vi "On Compile - Group Hardware Channels by Message Type.vi"(8 "error in":errorcluster, 11 "hardware channel data":T2[](array[typedef]) {"labels settings for RT"."Label Timestamp Channel Data Reference" format="%.0x"; "labels settings for RT"."Word Initial Raw Value" format="%032.0f"; "labels settings for RT"."Label Disable/Trigger Channel Reference" format="%.0x"; "labels settings for RT"."parameter driver data"."Tx parameter refs" format="%.0x"; "labels settings for RT"."SDI" format="%02b"; "labels settings for RT"."label" format="%.0o"}) -> (0 "error out":errorcluster, 3 "hardware channel data by transfer type":T10(array[cluster]) {"hardware channel data"."labels settings for RT"."Label Timestamp Channel Data Reference" format="%.0x"; "hardware channel data"."labels settings for RT"."Word Initial Raw Value" format="%032.0f"; "hardware channel data"."labels settings for RT"."Label Disable/Trigger Channel Reference" format="%.0x"; "hardware channel data"."labels settings for RT"."parameter driver data"."Tx parameter refs" format="%.0x"; "hardware channel data"."labels settings for RT"."SDI" format="%02b"; "hardware channel data"."labels settings for RT"."label" format="%.0o"; "Outgoing Channels" format="%.0x"; "ReadWrite Channels" format="%.0x"})   [LabVIEW 2020, in "AIM ARINC 429 System Explorer.lvlib" / "Implementation.lvlib"]
uses:
  Implementation.lvlib
  Shared/RT Hardware Channel Settings.ctl
  Shared/RT Label Settings.ctl
  Shared/Label.ctl
  Shared/RT Parameters.ctl
  Shared/Parameter Definition.ctl
  <vilib>/NI/NI VeriStand Encoding and Decoding/Encoding.ctl
  <vilib>/NI VeriStand/Custom Device API/Custom Device Item Ref.ctl
  Shared/Transfer Type.ctl
  <vilib>/NI VeriStand/Custom Device API/Data Reference.ctl
  <vilib>/NI VeriStand/Custom Device API/Custom Device API.lvlib
  <vilib>/NI/NI VeriStand Encoding and Decoding/Encoding and Decoding.lvlib
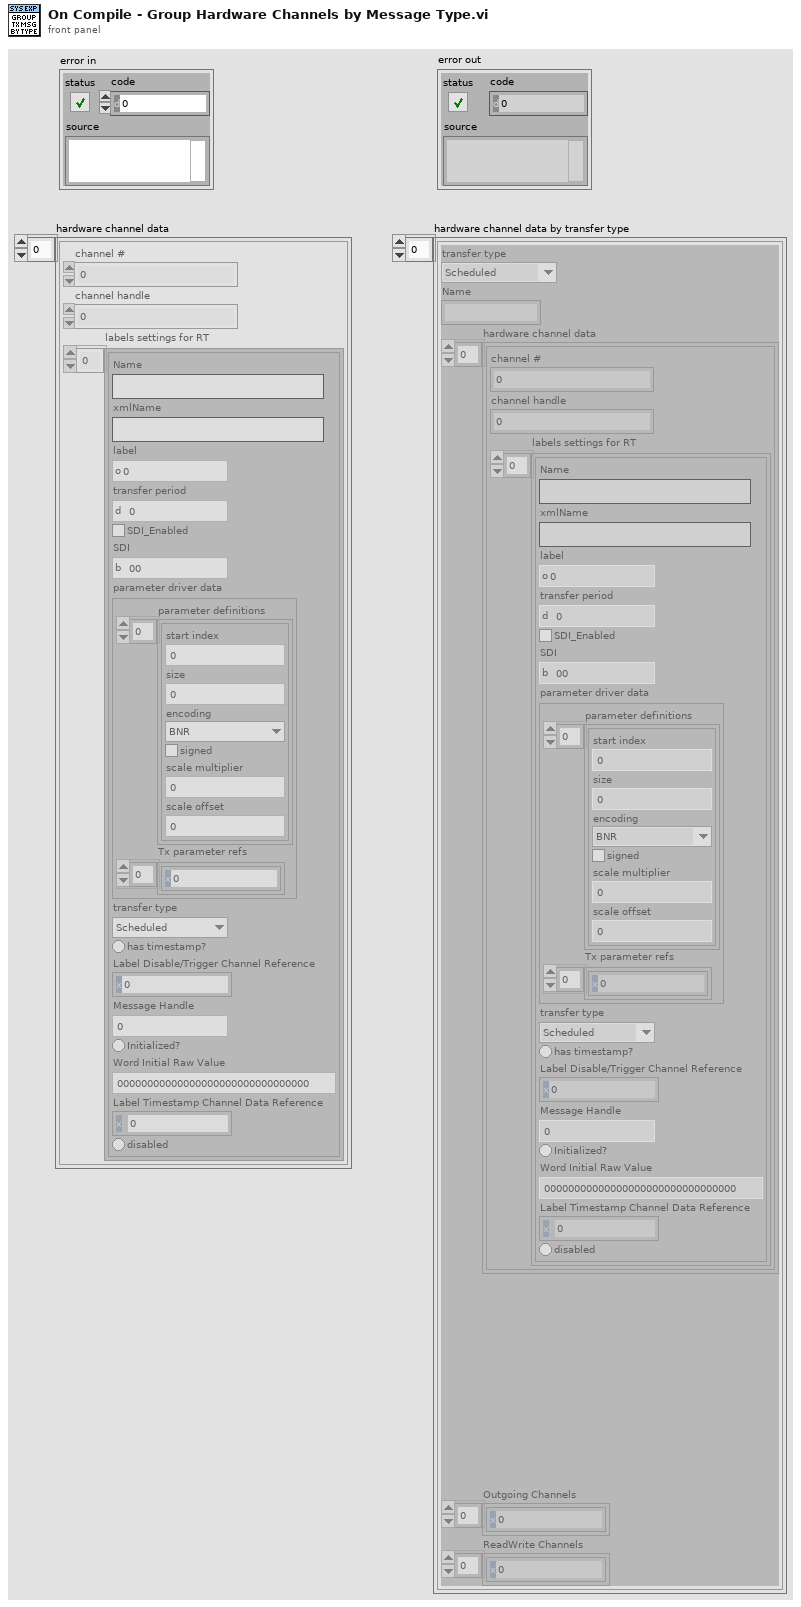
[diagram p1: front panel]
types:
  T1 = typedef "Transfer Type.ctl" = enum16{"Scheduled", "Acyclic", "Block", "Strobe"}
  T2 = typedef "RT Hardware Channel Settings.ctl" = cluster{"channel #":u16, "channel handle":u64, "labels settings for RT":T3[]}
  T3 = typedef "RT Label Settings.ctl" = cluster{"Name":string, "xmlName":string, "label":T4, "transfer period":u32, "SDI_Enabled":bool, "SDI":u8, "parameter driver data":T5, "transfer type":T1, "has timestamp?":bool, "Label Disable/Trigger Channel Reference":T8, "Message Handle":u64, "Initialized?":bool, "Word Initial Raw Value":u32, "Label Timestamp Channel Data Reference":T9, "disabled":bool}
  T4 = typedef "Label.ctl" = u8
  T5 = typedef "RT Parameters.ctl" = cluster{"parameter definitions":T6[], "Tx parameter refs":T8[]}
  T6 = typedef "Parameter Definition.ctl" = cluster{"start index":i32, "size":i32, "encoding":T7, "signed":bool, "scale multiplier":dbl, "scale offset":dbl}
  T7 = typedef "Encoding and Decoding.lvlib/Encoding.ctl" = enum16{"BNR", "BCD", "Discrete"}
  T8 = typedef "Custom Device API.lvlib/Custom Device Item Ref.ctl" = u64
  T9 = typedef "Custom Device API.lvlib/Data Reference.ctl" = i32
  T10 = cluster{"transfer type":T1, "Name":string, "hardware channel data":T2[], "Outgoing Channels":T8[], "ReadWrite Channels":T8[]}[]
  T11 = cluster{"transfer type":T1, "Name":string, "hardware channel data":T2[], "Outgoing Channels":T8[], "ReadWrite Channels":T8[]}
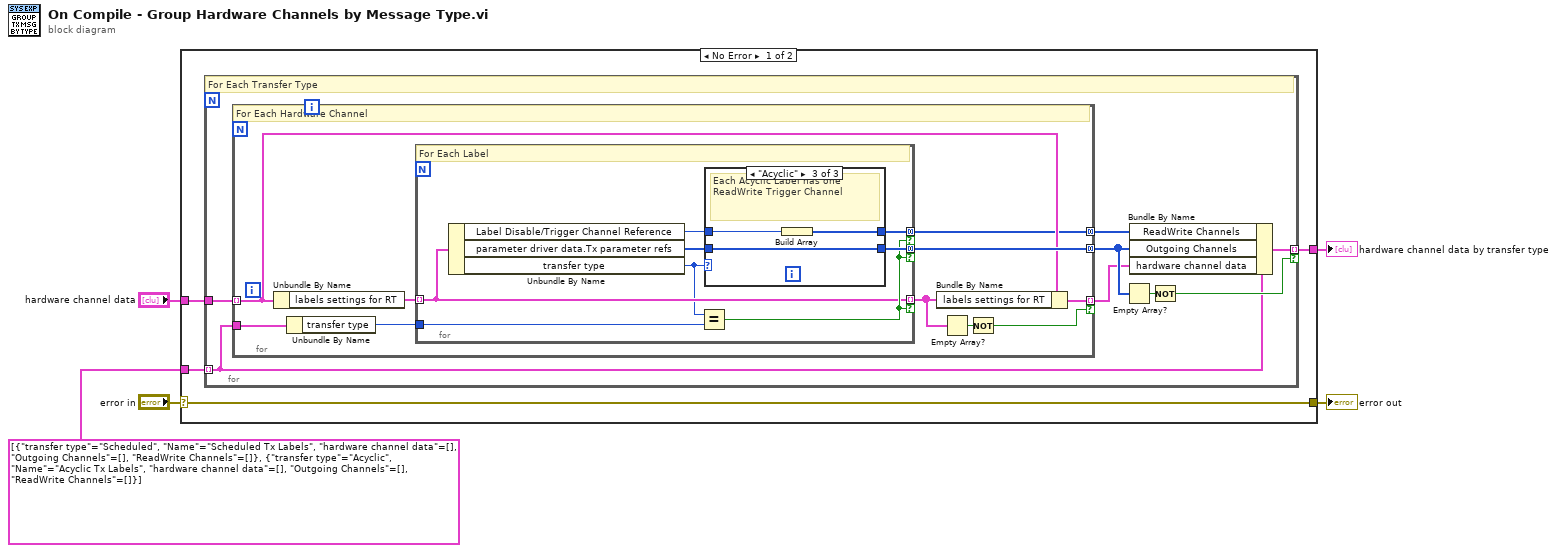
[diagram p0: block diagram]
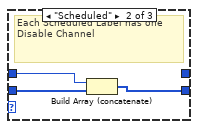
[diagram p3: hidden frame]
diagram:
  n1 = case shown="No Error" "error in" {
    selector: "error in" -> [w6 w42]
    tunnel: "hardware channel data" -> [w9 _]
    tunnel: [w6 w42] -> w3
    tunnel: T10 [{"transfer type"=enum."Scheduled", "Name"="Scheduled Tx Labels", "hardware channel data"=[], "Outgoing Channels"=[], "ReadWrite Channels"=[]}, {"transfer type"=enum."Acyclic", "Name"="Acyclic Tx Labels", "hardware channel data"=[], "Outgoing Channels"=[], "ReadWrite Channels"=[]}] -> [w8 _]
    tunnel: [w7 _] -> w2
    frame No Error {
      n2 = for {
        tunnel: w9 -> [w17]
        tunnel: w8 -> [w11] mode=indexing
        tunnel: [w16] -> w7 mode=indexing if=w14
        # "For Each Transfer Type"
        n3 = for {
          tunnel: w17 -> [w25] mode=indexing
          tunnel: [w26] -> w15 mode=concatenating
          tunnel: [w24] -> w10 mode=indexing if=w21
          tunnel: [w20] -> w13 mode=concatenating
          tunnel: w11 -> [w19]
          # "For Each Hardware Channel"
          n4 = Unbundle By Name(w25) -> ("labels settings for RT"=w27:T3[])
          n5 = Unbundle By Name(w19) -> ("transfer type"=w18:T1)
          n6 = for {
            tunnel: w27 -> [w29] mode=indexing
            tunnel: w18 -> [w30]
            tunnel: [w35] -> w26 mode=concatenating if=w31
            tunnel: [w29] -> w22 mode=indexing if=w31
            tunnel: [w32] -> w20 mode=concatenating if=w31
            # "For Each Label"
            n7 = Unbundle By Name(w29) -> ("Label Disable/Trigger Channel Reference"=w34:T8, "parameter driver data.Tx parameter refs"=w33:T8[], "transfer type"=w28:T1)
            n8 = Equal?(x=w28, y=w30) -> (x = y?=w31:bool)
            n9 = case shown="\"Acyclic\"" w28 {
              tunnel: [_ w37 w41] -> w35
              tunnel: w34 -> [_ w38 w40]
              tunnel: w33 -> [_ w36 w41]
              tunnel: [_ _ w39] -> w32
              frame Default {
                # "Unsupported Transfer Type"
              }
              frame "Scheduled" {
                # "Each Scheduled Label has one Disable Channel"
                n10 = Build Array (concatenate)(w38, w36) -> (w37:T8[])
              }
              frame "Acyclic" {
                # "Each Acyclic Label has one \nReadWrite Trigger Channel"
                n11 = Build Array(w40) -> (w39:T8[])
              }
            }
          }
          n12 = Bundle By Name(cluster=w25, "labels settings for RT"=w22) -> (w24:T2)
          n13 = Empty Array?(array=w22) -> (empty?=w23:bool)
          n14 = Not(x=w23) -> (.not. x?=w21:bool)
        }
        n15 = Empty Array?(array=w15) -> (empty?=w12:bool)
        n16 = Bundle By Name(cluster=w11, "ReadWrite Channels"=w13, "Outgoing Channels"=w15, "hardware channel data"=w10) -> (w16:T11)
        n17 = Not(x=w12) -> (.not. x?=w14:bool)
      }
    }
    frame Error {
    }
  }
  "error out" <- w3
  "hardware channel data by transfer type" <- w2
